vi "匹配字符串.vi"(11 "字符串":string="$GPRMC,014600.00,A,2237.496474,N,11356.089515,E,0.0,225.5,310518,2.3,W,A*23\r\n") -> (3 "所有匹配":string, 5 "是否匹配？":bool)   [LabVIEW 2016, in "GPS.lvlib" / "GPS.lvclass"]
uses:
  GPS.lvclass
  <vilib>/regexp/Match Regular Expression.xnode
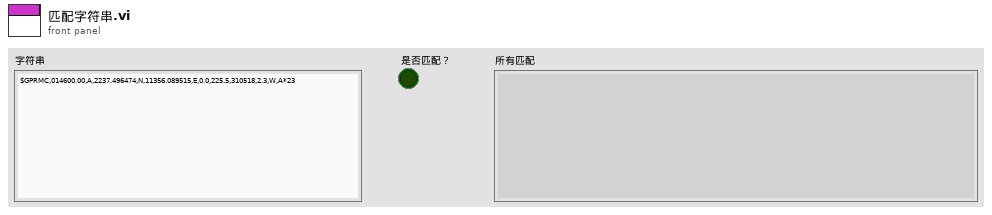
[diagram p1: front panel]
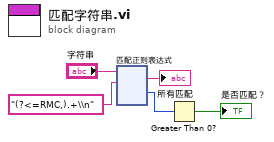
[diagram p0: block diagram]
diagram:
  n1 = xnode "匹配正则表达式"("输入字符串"="字符串", "正则表达式"="(?<=RMC,).+\\n") -> ("所有匹配"=→"所有匹配":string, "匹配后偏移量"=w2:i32)  [unwired: 4 in, 3 out]
  n2 = Greater Than 0?(x=w2) -> (x > 0?=→"是否匹配？":bool)
